vi "Overlay.vi"(8 "error in (no error)":errorcluster, 10 "Image In":T1, 11 "Overlay Base in":refnum<class "Analyze Results q-Factor.lvclass">) -> (0 "error out":errorcluster, 2 "Image out":T1, 3 "Overlay Base out":refnum<class "Analyze Results q-Factor.lvclass">)   [LabVIEW 2020, in "Analyze Results q-Factor.lvclass"]
uses:
  Analyze Results q-Factor.lvclass
  C:/POLARIS Programme/POLARIS-AS-3-Cams/Submodules/HIJ Vision/Analyze/Results and Overlays/Results Base/Analyze Results Base.lvclass
  <vilib>/vision/Image Controls.llb/IMAQ Image.ctl
  Results Base/Analyze Results Base.lvclass/Analyze Results Base.ctl
  Analyze Results q-Factor.lvclass/Analyze Results q-Factor.ctl
  Results Base/Read Overlay_.vi
  Read Focus ROI.vi
  Read q.vi
  Read Width Method.vi
  Read A.vi
  Results Base/Read Overlay colors.vi
  Results Base/Read Font, Size & Style.vi
  Results Base/Analyze Results Base.lvclass
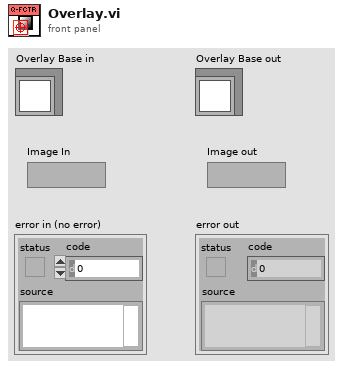
[diagram p1: front panel]
types:
  T1 = typedef "IMAQ Image.ctl" = refnum<image>
  T2 = typedef "ROI Descriptor" = cluster{"Global Rectangle":i32[], "Contours":cluster{"ID":enum32{"External", "Internal"}, "Type":u32, "Coordinates":i32[]}[]}
  T3 = cluster{"Desired Font (Application)":enum16{"User-specified Font", "Application Font", "System Font", "Dialog Font"}, "[User-specified Font]":cluster{"Font Name":string, "Size":i16, "Strikeout?":bool, "Italic?":bool, "Underline?":bool, "Outline?":bool, "Shadow?":bool, "Bold?":bool, "Rotation Angle":dbl}, "Horizontal Alignment":i16, "Vertical Alignment":i16}
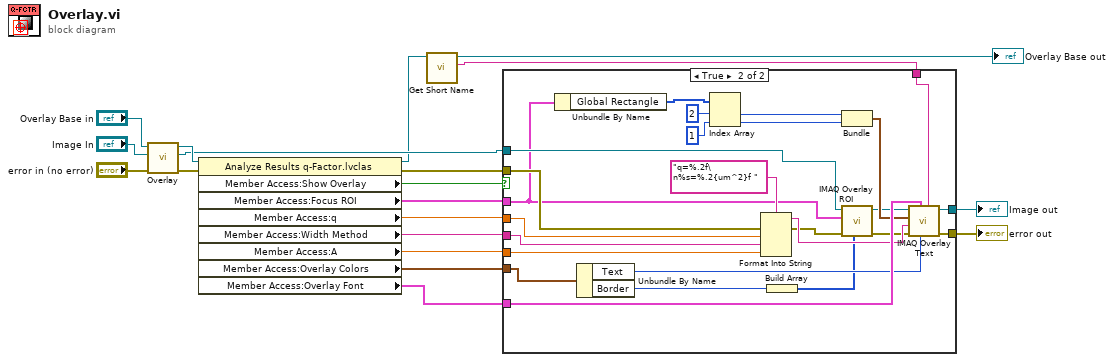
[diagram p0: block diagram]
diagram:
  n1 = call-parent "Overlay.vi"("error in (no error)"="error in (no error)", "Image In"="Image In", "Overlay Base in"="Overlay Base in") -> ("error out"=w14:errorcluster, "Image out"=w10:T1, "Overlay Base out"=w16:refnum<class "Analyze Results q-Factor.lvclass">)  [unwired: 6 in]
  n2 = property class="Analyze Results q-Factor.lvclas"(reference=w16, error in=w14) -> (reference out=w3:refnum<class "Analyze Results q-Factor.lvclass">, error out=w13:errorcluster, "Member Access:Show Overlay"=w15:bool, "Member Access:Focus ROI"=w9:T2, "Member Access:q"=w8:dbl, "Member Access:Width Method"=w7:string, "Member Access:A"=w6:dbl[unit], "Member Access:Overlay Colors"=w4:cluster{"Border":u32, "Text":u32}, "Member Access:Overlay Font"=w5:T3)
  n3 = call-dynamic "Get Short Name.vi"("Analyze Results Base in"=w3) -> ("Short Name"=w1:string, "Analyze Results Base out"=→"Overlay Base out":refnum<class "Analyze Results q-Factor.lvclass">)  [unwired: 8 in, 1 out]
  n4 = case shown="True" w15 {
    tunnel: w10 -> [w21 w40]
    tunnel: [w21 w44] -> w11
    tunnel: w13 -> [w20 w26]
    tunnel: [w20 w43] -> w12
    tunnel: w9 -> [_ w24]
    tunnel: w8 -> [_ w29]
    tunnel: w7 -> [_ w28]
    tunnel: w6 -> [_ w27]
    tunnel: w5 -> [_ w46]
    tunnel: w4 -> [_ w23]
    tunnel: w1 -> [_ w22]
    frame False {
    }
    frame True {
      n5 = Unbundle By Name(w24) -> ("Global Rectangle"=w34:i32[])
      n6 = Unbundle By Name(w23) -> ("Text"=w42:u32, "Border"=w38:u32)
      n7 = Index Array(array=w34, index #1=2 ("index"), index #2=1 ("index")) -> (element #1=w36:i32, element #2=w35:i32)
      n8 = Format Into String(format string="q=%.2f\n%s=%.2{um^2}f ", error in=w26, w29, w28, w27) -> (resulting string=w45:string, error out=w25:errorcluster)  [unwired: 1 in]
      n9 = Build Array(w38) -> (w37:u32[])
      n10 = Bundle(w36, w35) -> (w41:cluster{i32, i32})  [unwired: 1 in]
      n11 = call "IMAQ Overlay ROI"("Colors (Green)"=w37, "error in (no error)"=w25, "ROI Descriptor"=w24, "Image"=w40) -> ("error out"=w31:errorcluster, "Image Out"=w39:T1)  [unwired: 6 in]
      n12 = call "IMAQ Overlay Text"("Group"=w22, "Text Color (black)"=w42, "Font, Size & Style"=w46, "error in (no error)"=w31, "String"=w45, "Origin"=w41, "Image"=w39) -> ("error out"=w43:errorcluster, "Image Out"=w44:T1)  [unwired: 3 in]
    }
  }
  "error out" <- w12
  "Image out" <- w11
